vi "Torque Mode.vi"(8 "Fehler (Eingang, kein Fehler)":errorcluster) -> (0 "error out":errorcluster)   [LabVIEW 2014]
uses:
  <vilib>/CANopenLib/CANOPEN.llb/CANopen SDO Create.vi
  <vilib>/CANopenLib/CANOPEN.llb/CANopen SDO Write [I8].vi
  <vilib>/CANopenLib/CANOPEN.llb/CANopen SDO Write [U16].vi
  <vilib>/CANopenLib/CANOPEN.llb/CANopen SDO Close.vi
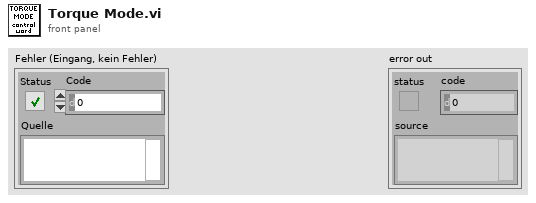
[diagram p1: front panel]
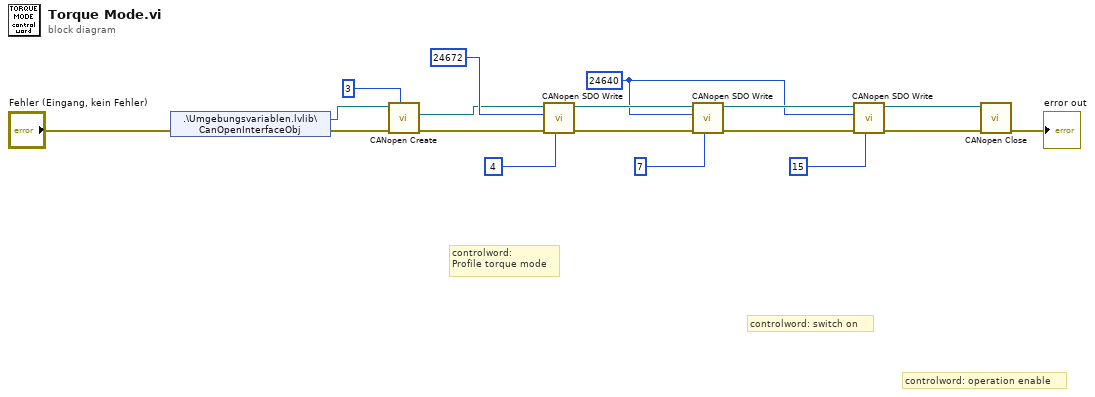
[diagram p0: block diagram]
diagram:
  w3 = u16 24640 ("object index")
  # "controlword: operation enable"
  # "controlword: switch on"
  # "controlword:\nProfile torque mode"
  n1 = shared-variable ".\\Umgebungsvariablen.lvlib\\CanOpenInterfaceObj"(error in="Fehler (Eingang, kein Fehler)") -> (w17:refnum<k20>, error out=w18:errorcluster)
  n2 = call-poly <vilib>:"CANopen Create.vi"("node-ID"=u8 3, "error in (no error)"=w18, "interface object in"=w17) -> ("error out"=w12:errorcluster, "SDO object out"=w13:refnum<k20>)  [unwired: 6 in, 1 out]
  n3 = call-poly <vilib>:"CANopen SDO Write.vi"("I8 data"=i8 4, "error in (no error)"=w12, "object index"=u16 24672, "SDO object in"=w13) -> ("error out"=w6:errorcluster, "SDO object out"=w7:refnum<k20>)  [unwired: 5 in, 1 out]
  n4 = call-poly <vilib>:"CANopen SDO Write.vi"("U16 data"=u16 7, "error in (no error)"=w6, "object index"=w3, "SDO object in"=w7) -> ("error out"=w4:errorcluster, "SDO object out"=w5:refnum<k20>)  [unwired: 5 in, 1 out]
  n5 = call-poly <vilib>:"CANopen SDO Write.vi"("U16 data"=u16 15, "error in (no error)"=w4, "object index"=w3, "SDO object in"=w5) -> ("error out"=w1:errorcluster, "SDO object out"=w2:refnum<k20>)  [unwired: 5 in, 1 out]
  n6 = call-poly <vilib>:"CANopen Close.vi"("error in (no error)"=w1, "SDO object in"=w2) -> ("error out"=→"error out":errorcluster)  [unwired: 9 in]
